vi "Open.vi"(0 "file path":path, 1 "sample rate (SPS)":dbl, 2 "block duration (s) (0.01)":dbl=0.01, 3 "I/O mode (Data Reference)":T1=enum."Data Reference", 4 "disable buffering? (T)":bool=TRUE, 5 "error in (no error)":errorcluster, 6 "disk read (F) / write (T)":bool, 7 "# of blocks (5)":u32=5) -> (14 "disk streaming out":refnum<class "Disk Streaming.lvclass">, 15 "host DMA buffer size (samples)":u32, 16 "host DMA buffer num of blocks":u32, 17 "host DMA buffer block size divisor (bytes)":u32, 19 "error out":errorcluster)   [LabVIEW 2021, in "Disk Streaming.lvclass"]
doc: "Opens a TDMS file and creates a disk streaming instance referencing the file for streaming samples between a disk and an FPGA Target. Once the instance is created, use the <B>Configure.vi</B> to configure the transfer. Use the <B>Get Next Transfer Size.vi</B> to get the size of the next block to transfer during the streaming process, then depending on the selected direction and the TDMS I/O functions, use the <B>Read (I16 Data Ref).vi</B>, <B>Read (I16).vi</B>, <B>Write (I16 Data Ref).vi</B> or <B>Write (I16).vi</B> to read or write the TDMS file. Use the <B>Configure Status.vi</B> to configure the streaming status properties. Use the <B>Get Status.vi</B> to get status information. Use the <B>Close.vi</B> to close the disk streaming instance and the TDMS file it uses.\n\nInputs:\n\n<B>file path</B>: The absolute path to the TDMS file to open for the streaming. When streaming to disk, this file is written with the samples streamed from the FPGA Target. When streaming from disk, the contents of this file are streamed to the FPGA Target.\n\n<B>sample rate (SPS)</B>: The expected sample rate of the stream.\n\n<B>block duration (s)</B>: The desired time duration, in seconds, covered by each block transferred during the streaming. The desired size of each block is <B>block duration (s)</B> * <B>sample rate (SPS)</B> samples. The default value of this input is 0.01, which specifies a duration of 10ms.\n\n<B>I/O mode</B>: Selects the TDMS I/O functions to use during the streaming. Set this input to \"Data Reference\" to use the TDMS Advanced Data Reference I/O functions during the streaming: in this case use the <B>Write (I16 Data Ref).vi</B> or the <B>Read (I16 Data Ref).vi</B> to write or read the TDMS file, which functions require an External Data Value Reference (EDVR) referencing the I16 array to write to the file or to write with the samples read from the file. Set this input to \"Synchronous\" or \"Asynchronous\" to use the TDMS Advanced Synchronous I/O functions or the TDMS Advanced Asynchronous I/O functions, respectively, during the streaming: in these cases use the <B>Write (I16).vi</B> or the <B>Read (I16).vi</B> to write or read the TDMS file, which functions expect the samples to write to the file or return the samples read from the file in an array of I16s. The default value of this input is \"Data Reference\".\n\n<B>disable buffering?</B>: Specifies whether to open the TDMS file without system buffering. Disabling system buffering can speed up data transfers in certain situations. If you have a small amount of data to transfer, you might not notice a difference if you disable buffering. To read or write a data file to a Redundant Array of Independent Disks (RAID), consider opening the file without buffering to speed up data transfers. To read the same set of data repeatedly from the computer, consider enabling buffering. The default value of this input is true.\n\n<B>disk read (F) / write (T)</B>: Specifies the stream direction: when true, the TDMS file is written (stream to disk); when false, the TDMS file is read (stream from disk).\n\n<B># of blocks</B>: The number of blocks the host DMA buffer size should be configured for. This input is coerced to be at least 2. The default value of this input is 5.\n\nOutputs:\n\n<B>disk streaming out</B>: Disk streaming instance output. Pass this output to the other Disk Streaming VIs to perform the streaming.\n\n<B>host DMA buffer size (samples)</B>: The minimum required host DMA buffer size, given in number of samples. When streaming between a disk and an FPGA Target, configure the size of the host FIFO of the DMA channel transferring the samples between the host and the FPGA Target to be large enough to hold at least as many samples as the value returned on this output.\n\n<B>host DMA buffer num of blocks</B>, <B>host DMA buffer block size divisor (bytes)</B>: Host DMA buffer size constraints. When streaming between a disk and an FPGA Target, configure the size of the host FIFO of the DMA channel transferring the samples between the host and the FPGA Target to be a multiple of <B>host DMA buffer num of blocks</B>, and dividing the size of the allocated host DMA buffer by <B>host DMA buffer num of blocks</B> should result in a size which is an integer multiple of the sample size, and in bytes is an integer multiple of the <B>host DMA buffer block size divisor (bytes)</B>. Refer to the <B>Example - Configure Host DMA Buffer Size.vi</B> for an example on how to configure the host DMA buffer size to fulfill these requirements."
uses:
  Disk Streaming.lvclass
  IO mode.ctl
  Private/Data.ctl
  Private/Command.ctl
  Private/Status.ctl
  Disk Streaming.lvclass/Disk Streaming.ctl
  kernel32.dll
  <vilib>/gmath/NI_Gmath.lvlib
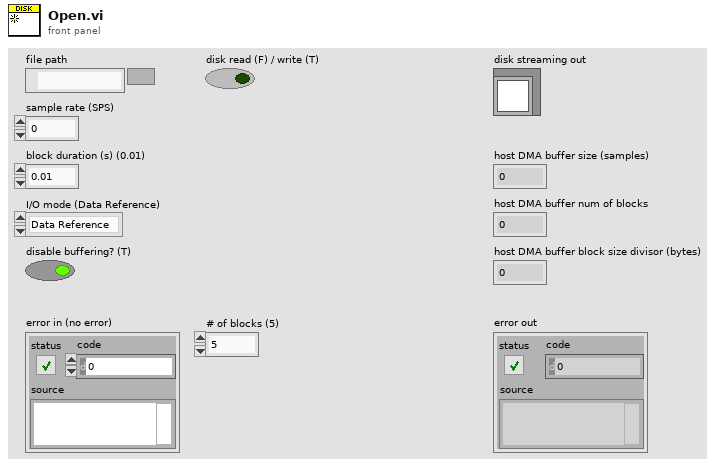
[diagram p1: front panel]
types:
  T1 = typedef "Disk Streaming.lvclass/IO mode.ctl" = enum16{"Synchronous", "Asynchronous", "Data Reference"}
  T2 = typedef "Disk Streaming.lvclass/Status.ctl" = cluster{"finished":bool, "Host DMA buffer size (bytes)":u64, "Host DMA buffer utilization (bytes)":u64, "Disk maximum async operations":u32, "Disk pending async operations":u32, "preview data":i16[]}
  T3 = typedef "Disk Streaming.lvclass/Command.ctl" = cluster{"preview size":i32}
  T4 = typedef "Disk Streaming.lvclass/Data.ctl" = cluster{"tdms file":refnum<k34>, "group name":string, "channel name":string, "max operations":u32, "timeout (s)":dbl, "data type size (bytes)":u64, "writing":bool, "I/O mode":T1, "# of blocks":u32, "block size divisor (bytes)":u32, "file position (elements)":u64, "file size (elements)":i64, "file size (samples)":i64, "block size (elements)":u64, "block size (samples)":u64, "quantum size (elements)":u64, "quantum size (samples)":u64, "samples remaining":i64, "elements transferred":u64, "finished":bool, "preview size":i32, "preview quantum size (elements)":u64, "preview quantum size (samples)":u64, "DMA buffer size (elements)":u32, "pending block sizes (bytes)":u64[]}
  T5 = enum16{"open", "open or create", "create or replace", "create", "open (read-only)"}
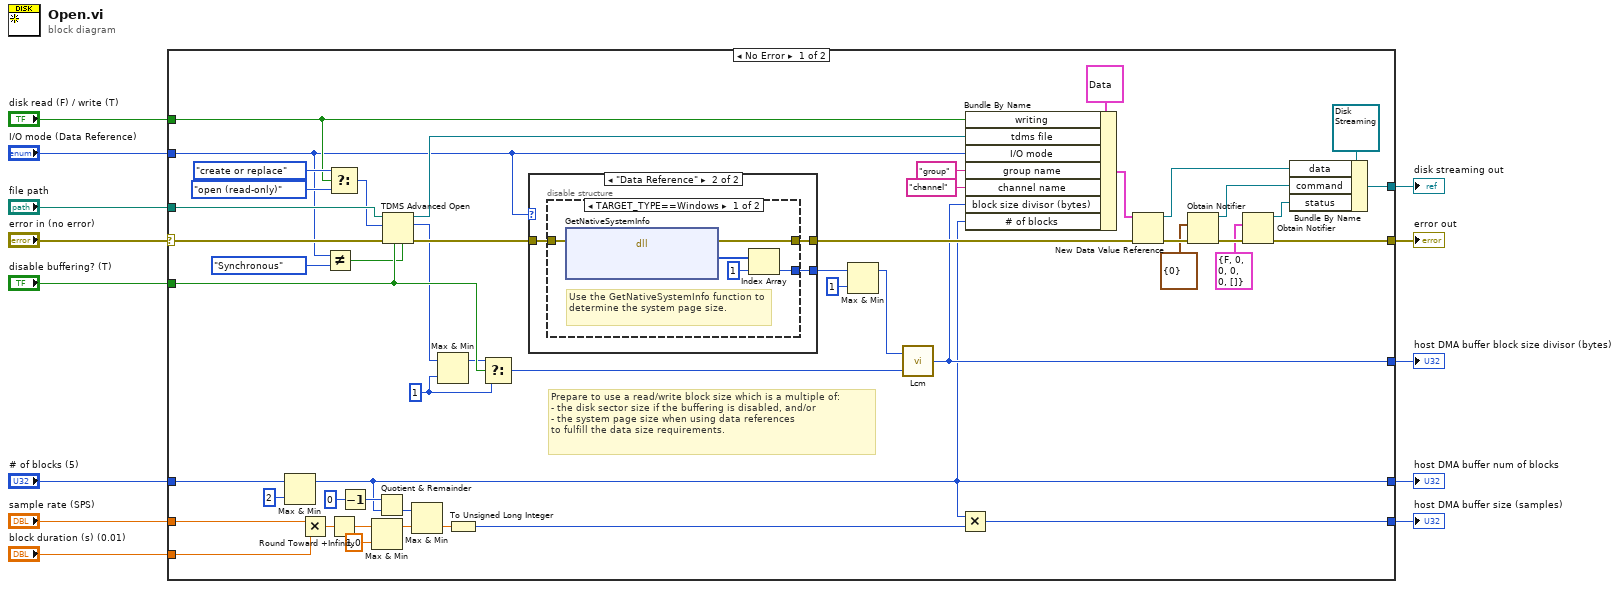
[diagram p0: block diagram]
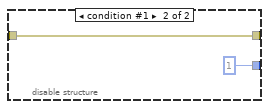
[diagram p3: hidden frame]
diagram:
  n1 = case shown="No Error" "error in (no error)" {
    selector: "error in (no error)" -> [w63 w75]
    tunnel: [w22 w75] -> w12
    tunnel: "file path" -> [w60 _]
    tunnel: "# of blocks (5)" -> [w33 _]
    tunnel: "block duration (s) (0.01)" -> [w58 _]
    tunnel: "sample rate (SPS)" -> [w59 _]
    tunnel: [w55 _] -> w7
    tunnel: "disable buffering? (T)" -> [w45 _]
    tunnel: "I/O mode (Data Reference)" -> [w15 _]
    tunnel: "disk read (F) / write (T)" -> [w35 _]
    tunnel: [w21 _] -> w4
    tunnel: [w18 _] -> w2
    tunnel: [w17 _] -> w1
    frame No Error {
      w42 = u32 1 ("y")
      # "Prepare to use a read/write block size which is a multiple of:\n- the disk sector size if the buffering is disabled, and/or\n- the system page size when using data references\nto fulfill the data size requirements."
      n2 = Max & Min(x=w33, y=u32 2) -> (max(x,y)=w17:u32)  [unwired: 1 out]
      n3 = Multiply(x=w59, y=w58) -> (x*y=w57:dbl)
      n4 = Not Equal?(x=w15, y=IO_mode."Synchronous") -> (x != y?=w16:bool)
      n5 = Select(t=T5."create or replace" ("operation (0:open)"), s=w35, f=T5."open (read-only)") -> (s? t:f=w36:T5)
      n6 = Round Toward +Infinity(x=w57) -> (ceil(x): smallest int >= x=w48:dbl)
      n7 = Decrement(x=u32 0) -> (x-1=w52:u32)
      n8 = Max & Min(x=w48, y=1.0) -> (max(x,y)=w47:dbl)  [unwired: 1 out]
      n9 = Quotient & Remainder(x=w52, y=w17) -> (floor(x/y)=w51:u32)  [unwired: 1 out]
      n10 = TDMS Advanced Open(4:w16, 6:w45, 8:w63, 10:w36, 11:w60) -> (0:w62:errorcluster, 2:w34:u32, 3:w54:refnum<k34>)
      n11 = Max & Min(x=w51, y=w47) -> (min(x,y)=w50:dbl)  [unwired: 1 out]
      n12 = Max & Min(x=w34, y=w42) -> (max(x,y)=w44:u32)  [unwired: 1 out]
      n13 = To Unsigned Long Integer(number=w50) -> (unsigned 32bit integer=w56:u32)
      n14 = Select(t=w44, s=w45, f=w42) -> (s? t:f=w43:u32)
      n15 = case shown="\"Data Reference\"" w15 {
        tunnel: w62 -> [w64 w67]
        tunnel: [w64 w66] -> w61
        tunnel: [_ w65] -> w41
        frame Default {
        }
        frame "Data Reference" {
          n16 = disable-structure shown="TARGET_TYPE==Windows" {
            disable-tunnel: [w69 w74] -> w66
            disable-tunnel: [w70 u32 1] -> w65
            disable-tunnel: w67 -> [w68 w74]
            frame condition #0 (active) {
              # "Use the GetNativeSystemInfo function to determine the system page size."
              n17 = dll-call lib="kernel32.dll" fn="GetNativeSystemInfo"(error in=w68) -> (error out=w69:errorcluster, "lpSystemInfo"=w71:u32[])  [unwired: 4 in, 1 out]
              n18 = Index Array(array=w71, index=1) -> (element=w70:u32)
            }
            frame condition #1 {
            }
          }
        }
      }
      n19 = Max & Min(x=w41, y=u32 1) -> (max(x,y)=w39:u32)  [unwired: 1 out]
      n20 = call <vilib>:"Lcm.vi"("y"=w43, "x"=w39) -> ("lcm(x,y)"=w18:i64)
      n21 = Multiply(x=w17, y=w56) -> (x*y=w55:u32)
      n22 = Bundle By Name(cluster=T4 {"tdms file"=refnum, "group name"="", "channel name"="", "max operations"=0, "timeout (s)"=0.0, "data type size (bytes)"=0, "writing"=FALSE, "I/O mode"=enum."Synchronous", "# of blocks"=0, "block size divisor (bytes)"=0, "file position (elements)"=0, "file size (elements)"=0, "file size (samples)"=0, "block size (elements)"=0, "block size (samples)"=0, "quantum size (elements)"=0, "quantum size (samples)"=0, "samples remaining"=0, "elements transferred"=0, "finished"=FALSE, "preview size"=0, "preview quantum size (elements)"=0, "preview quantum size (samples)"=0, "DMA buffer size (elements)"=0, "pending block sizes (bytes)"=[]} ("Disk Streaming Descriptor Data"), "writing"=w35, "tdms file"=w54, "I/O mode"=w15, "group name"="group", "channel name"="channel", "block size divisor (bytes)"=w18, "# of blocks"=w17) -> (w53:T4)
      n23 = New Data Value Reference(data value=w53, error in=w61) -> (data value reference=w28:refnum<data-value>, error out=w30:errorcluster)
      n24 = Obtain Notifier(notification data type=T3 {"preview size"=0} ("Disk Streaming Descriptor Command"), error in (no error)=w30) -> (notifier out=w26:refnum<notifier>, error out=w25:errorcluster)  [unwired: 2 in, 1 out]
      n25 = Obtain Notifier(notification data type=T2 {"finished"=FALSE, "Host DMA buffer size (bytes)"=0, "Host DMA buffer utilization (bytes)"=0, "Disk maximum async operations"=0, "Disk pending async operations"=0, "preview data"=[]} ("Disk Streaming Descriptor Status"), error in (no error)=w25) -> (notifier out=w23:refnum<notifier>, error out=w22:errorcluster)  [unwired: 2 in, 1 out]
      n26 = Bundle By Name(cluster=refnum<class "Disk Streaming.lvclass"> refnum ("Disk Streaming.lvclass"), "data"=w28, "command"=w26, "status"=w23) -> (w21:refnum<class "Disk Streaming.lvclass">)
    }
    frame Error {
    }
  }
  "error out" <- w12
  "host DMA buffer size (samples)" <- w7
  "disk streaming out" <- w4
  "host DMA buffer block size divisor (bytes)" <- w2
  "host DMA buffer num of blocks" <- w1
